vi "MyClass1_IMyInterface_Create.vi"(0 "reference in":refnum<class "G#Object.lvclass">, 5 "error in (no error)":errorcluster) -> (14 "reference out":refnum<class "MyClass1_IMyInterface.lvclass">, 19 "error out":errorcluster)   [LabVIEW 2017, in "MyClass1_IMyInterface.lvclass"]
doc: "Creates the interface for the G#Object."
uses:
  MyClass1_IMyInterface.lvclass
  C:/Projects/GsharpGIT/G# Framework/examples/AddQ/G#/Interface/IMyInterface_interface/IMyInterface.lvclass
  <vilib>/addons/_AddQ/G#Object/G#Object.lvclass
  IMyInterface_interface/IMyInterface.lvclass
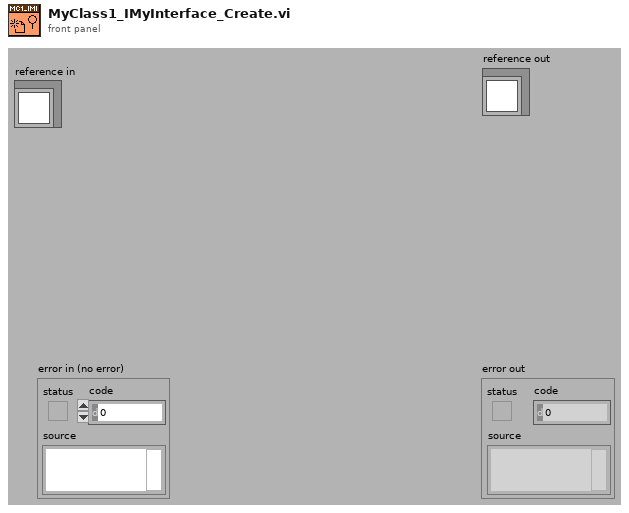
[diagram p1: front panel]
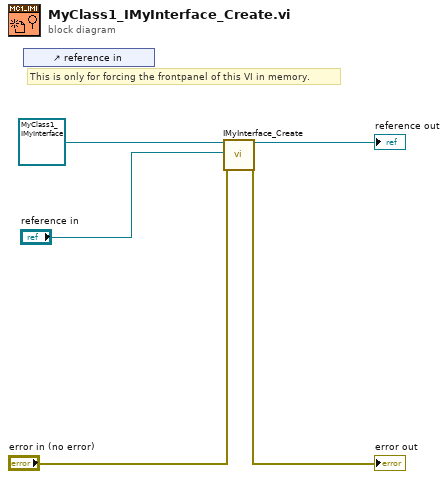
[diagram p0: block diagram]
diagram:
  # "This is only for forcing the frontpanel of this VI in memory."
  n1 = control-ref of="reference in"() -> ()  [unwired: 1 out]
  n2 = call "IMyInterface_Create.vi"("reference in"=refnum<class "MyClass1_IMyInterface.lvclass"> refnum ("reference out"), "G#Object in"="reference in", "error in (no error)"="error in (no error)") -> ("reference out"=→"reference out":refnum<class "MyClass1_IMyInterface.lvclass">, "error out"=→"error out":errorcluster)  [unwired: 15 in]
